vi "Simple FPGA Personality.vi"() -> ()   [LabVIEW 2018]
uses:
  Speciality IO/Types/Static.Generate.Digital.Settings.ctl
  Speciality IO/Types/Static.Measure.Digital.Measurement.ctl
  <vilib>/rvi/Emulation/niFpgaGetClockAttributes.vi
  <vilib>/rvi/Emulation/niFpgaSctlEmulationGetInTimedLoop.vi
  <vilib>/rvi/Emulation/niFpgaEmulationReportErrorSimple.vi
  <vilib>/rvi/Emulation/niFpgaCriticalErrorInLSC.vi
  Speciality IO/Speciality FPGA IO.lvlib
panel:
  out "Measurement":T1
  in  "Settings":T2={"ACTIVE EDGE"=TRUE, "OUTPUT"=FALSE}
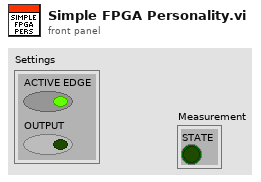
[diagram p1: front panel]
types:
  T1 = typedef "Speciality FPGA IO.lvlib/Static.Measure.Digital.Measurement.ctl" = cluster{"STATE":bool}
  T2 = typedef "Speciality FPGA IO.lvlib/Static.Generate.Digital.Settings.ctl" = cluster{"ACTIVE EDGE":bool, "OUTPUT":bool}
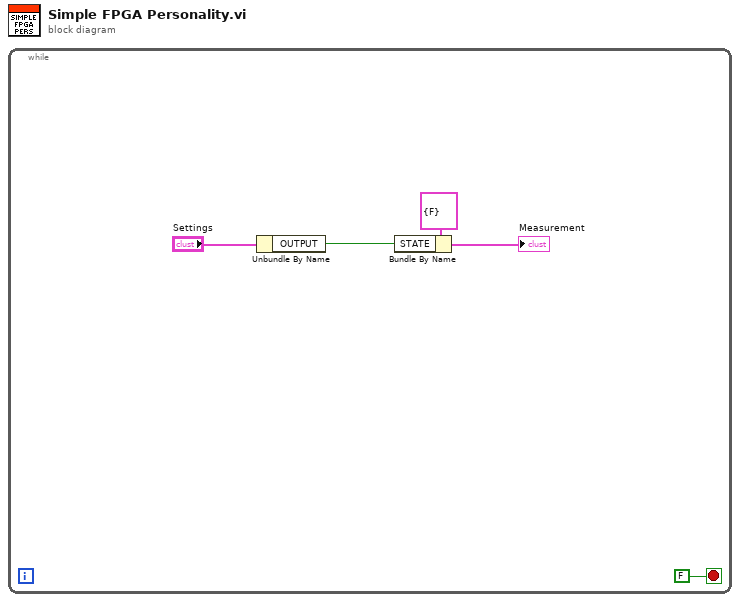
[diagram p0: block diagram]
diagram:
  n1 = while {
    stop <- FALSE stop-if-true
    n2 = Unbundle By Name("Settings") -> ("OUTPUT"=w2:bool)
    n3 = Bundle By Name(cluster=T1 {"STATE"=FALSE} ("Measurement"), "STATE"=w2) -> (→"Measurement":T1)
  }
